vi "ActionVIOnCompile.vi"(8 "error in (no error)":errorcluster, 11 "Device Item Ref in":T1 format="%.0x") -> (0 "error out":errorcluster)   [LabVIEW 2017, in "VeriStand Web Service Demo System Explorer.lvlib"]
uses:
  VeriStand Web Service Demo System Explorer.lvlib
  <vilib>/NI Veristand/Custom Device API/Custom Device Item Ref.ctl
  Shared/Compiled.Settings.ctl
  <vilib>/NI/NI VeriStand Advanced SysDef API/_SubVIs/SysDef.Property.Get.String.vi
  <vilib>/NI Veristand/Custom Device Tools/Custom Device Utility Library/NI VeriStand - Search for Item by Name.vi
  <vilib>/NI Veristand/Custom Device API/Set Item Property (Variant).vi
  <vilib>/NI VeriStand/Custom Device Tools/Custom Device Utility Library/Custom Device Utility Library.lvlib
  <vilib>/NI Veristand/Custom Device API/Custom Device API.lvlib
  <vilib>/NI/NIVS Inline Async API/_Data Access System Explorer/Data Access System Explorer.lvlib
  Shared/VeriStand Web Service Demo Shared.lvlib
  <vilib>/NI/NI VeriStand Advanced SysDef API/SysDef API/Advanced System Definition.lvlib
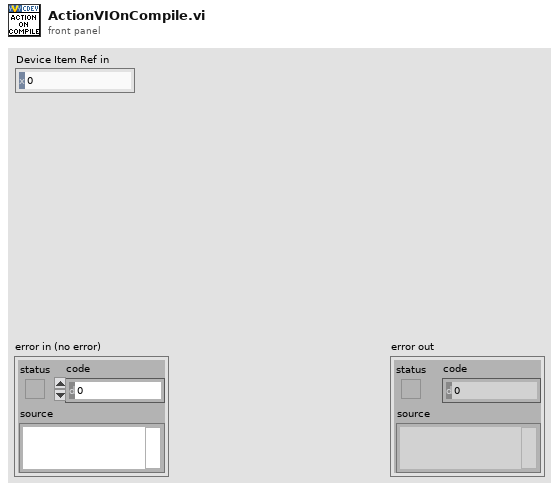
[diagram p1: front panel]
types:
  T1 = typedef "Custom Device API.lvlib/Custom Device Item Ref.ctl" = u64
  T2 = typedef "VeriStand Web Service Demo Shared.lvlib/Compiled.Settings.ctl" = cluster{"queueName":string}
  T3 = cluster{"Name":string, "Type":enum16{"Output/Write", "Input/Read", "Input/ReadWrite"}, "VS Refs":T1[]}
  T4 = enum16{"Output/Write", "Input/Read", "Input/ReadWrite"}
  T5 = cluster{"Name":string, "Type":enum16{"Output/Write", "Input/Read", "Input/ReadWrite"}, "VS Refs":T1[]}[]
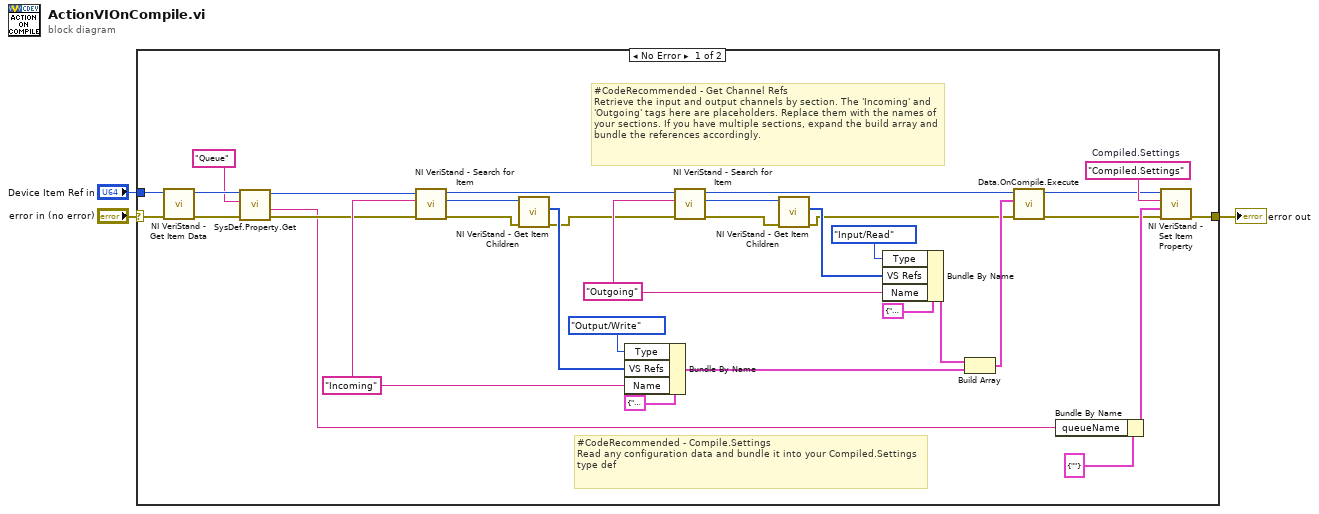
[diagram p0: block diagram]
diagram:
  n1 = case shown="No Error" "error in (no error)" {
    selector: "error in (no error)" -> [w29 w37]
    tunnel: [w30 w37] -> w2
    tunnel: "Device Item Ref in" -> [w28 _]
    frame No Error {
      w25 = "Outgoing" ("Item Name")
      w27 = "Incoming" ("Item Name")
      w32 = "Compiled.Settings"  # Compiled.Settings
      # "#CodeRecommended - Get Channel Refs\nRetrieve the input and output channels by section. The 'Incoming' and 'Outgoing' tags here are placeholders. Replace them with the names of your sections. If you have multiple sections, expand the build array and bundle the references accordingly."
      # "#CodeRecommended - Compile.Settings\nRead any configuration data and bundle it into your Compiled.Settings type def"
      n2 = call <vilib>:"NI VeriStand - Get Item Data.vi"("error in (no error)"=w29, "Item Ref in"=w28) -> ("error out"=w8:errorcluster, "Item Ref out"=w9:T1)  [unwired: 6 in, 2 out]
      n3 = call-poly <vilib>:"SysDef.Property.Get.vi"("error in (no error)"=w8, "Property Name"="Queue", "nodeID"=w9) -> ("error out"=w6:errorcluster, "Value out"=w4:string, "nodeID out"=w7:u64)  [unwired: 5 in, 1 out]
      n4 = call-poly <vilib>:"NI VeriStand - Search for Item.vi"("error in"=w6, "Item Name"=w27, "Section Ref in"=w7) -> ("error out"=w36:errorcluster, "Item Ref"=w35:T1, "Section Ref out"=w14:T1)  [unwired: 5 in, 1 out]
      n5 = call <vilib>:"NI VeriStand - Get Item Children.vi"("error in (no error)"=w36, "Item Ref in"=w35) -> ("error out"=w13:errorcluster, "Child Refs"=w26:T1[])  [unwired: 6 in, 2 out]
      n6 = Bundle By Name(cluster=T3 {"Name"="", "Type"=enum."Output/Write", "VS Refs"=[]} ("Group"), "Type"=T4."Output/Write", "VS Refs"=w26, "Name"=w27) -> (w17:T3)
      n7 = call-poly <vilib>:"NI VeriStand - Search for Item.vi"("error in"=w13, "Item Name"=w25, "Section Ref in"=w14) -> ("error out"=w33:errorcluster, "Item Ref"=w34:T1, "Section Ref out"=w15:T1)  [unwired: 5 in, 1 out]
      n8 = call <vilib>:"NI VeriStand - Get Item Children.vi"("error in (no error)"=w33, "Item Ref in"=w34) -> ("error out"=w16:errorcluster, "Child Refs"=w21:T1[])  [unwired: 6 in, 2 out]
      n9 = Bundle By Name(cluster=T3 {"Name"="", "Type"=enum."Output/Write", "VS Refs"=[]} ("Group"), "Type"=T4."Input/Read", "VS Refs"=w21, "Name"=w25) -> (w23:T3)
      n10 = Build Array(w23, w17) -> (w20:T5)
      n11 = call <vilib>:"Data.OnCompile.Execute.vi"("error in"=w16, "VS Ref Groups"=w20, "Custom Device Ref"=w15) -> ("error out"=w12:errorcluster, "Custom Device Ref"=w11:T1)  [unwired: 7 in]
      n12 = Bundle By Name(cluster=T2 {"queueName"=""} ("Compiled.Settings"), "queueName"=w4) -> (w31:T2)
      n13 = call-poly <vilib>:"NI VeriStand - Set Item Property.vi"("error in (no error)"=w12, "Value"=w31, "Property Name"=w32, "Item Ref in"=w11) -> ("error out"=w30:errorcluster)  [unwired: 5 in, 2 out]
    }
    frame Error {
    }
  }
  "error out" <- w2
